vi "Array to File.vi"(8 "error in":errorcluster, 10 "array in":T1[](array[typedef]) {"Last Updated" format="%<%x>T"}, 11 "file path in":path) -> (0 "error out":errorcluster, 3 "file path out":path)   [LabVIEW 2018]
uses:
  SR Cluster.ctl
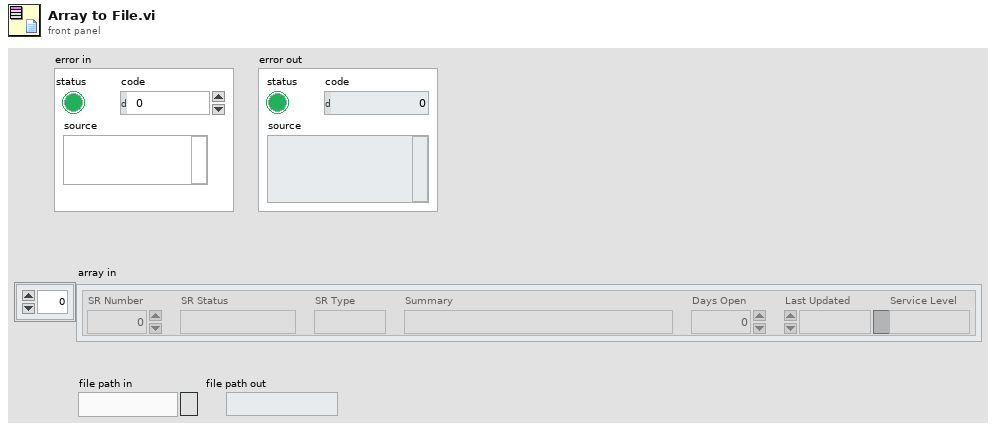
[diagram p1: front panel]
types:
  T1 = typedef "SR Cluster.ctl" = cluster{"SR Number":i32, "SR Status":string, "SR Type":string, "Summary":string, "Days Open":dbl, "Last Updated":timestamp, "Service Level":string}
  T2 = enum16{"open", "replace", "create", "open or create", "replace or create", "replace or create with confirmation"}
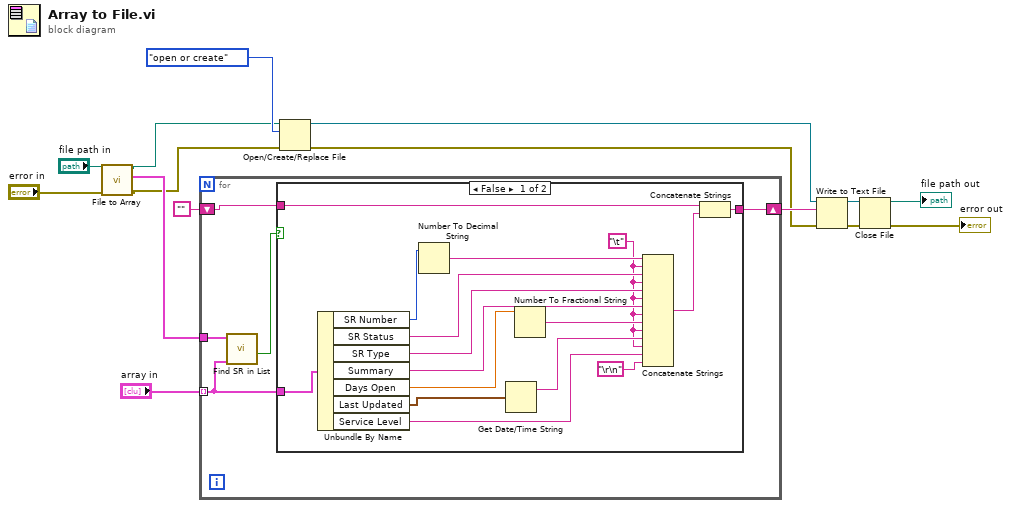
[diagram p0: block diagram]
diagram:
  n1 = call "File to Array.vi"("error in"="error in", "file path in"="file path in") -> ("error out"=w2:errorcluster, "list out"=w3:T1[], "file path out"=w4:path)  [unwired: 7 in]
  n2 = for {
    tunnel: "array in" -> [w16] mode=indexing
    tunnel: w3 -> [w18]
    shift-right: [w20] -> w12
    shift-left: "" -> [w19]
    n3 = call "Find SR in List.vi"("new SR"=w16, "SR list in"=w18) -> ("Is SR in List?"=w17:bool)  [unwired: 8 in, 1 out]
    n4 = case shown="False" w17 {
      tunnel: [w36 w37] -> w20
      tunnel: w19 -> [w35 w37]
      tunnel: w16 -> [w33 _]
      frame False {
        w22 = "\t"
        n5 = Unbundle By Name(w33) -> ("SR Number"=w32:i32, "SR Status"=w30:string, "SR Type"=w29:string, "Summary"=w23:string, "Days Open"=w28:dbl, "Last Updated"=w24:timestamp, "Service Level"=w25:string)
        n6 = Number To Decimal String(number=w32) -> (decimal integer string=w31:string)  [unwired: 1 in]
        n7 = Get Date/Time String(seconds (now)=w24) -> (date string=w26:string)  [unwired: 2 in, 1 out]
        n8 = Number To Fractional String(number=w28) -> (F-format string=w27:string)  [unwired: 3 in]
        n9 = Concatenate Strings(w31, w22, w30, w22, w29, w22, w23, w22, w27, w22, w26, w22, w25, "\r\n") -> (w34:string)
        n10 = Concatenate Strings(w35, w34) -> (w36:string)
      }
      frame True {
      }
    }
  }
  n11 = Open/Create/Replace File(file path (use dialog)=w4, error in=w2, operation (0:open)=T2."open or create") -> (refnum out=w10:refnum<file>, error out=w11:errorcluster)  [unwired: 3 in, 1 out]
  n12 = Write to Text File(file (use dialog)=w10, text=w12, error in=w11) -> (refnum out=w8:refnum<file>, error out=w9:errorcluster)  [unwired: 1 in, 1 out]
  n13 = Close File(refnum=w8, error in=w9) -> (path=→"file path out":path, error out=→"error out":errorcluster)
